vi "Read productId.vi"(8 "error in (no error)":errorcluster, 11 "SCD in":refnum<class "SCD.lvclass">) -> (0 "error out":errorcluster, 2 "productId":i32, 3 "SCD out":refnum<class "SCD.lvclass">)   [LabVIEW 2023, in "SCD.lvclass"]
uses:
  SCD.lvclass
  GenericDevice/GenericDevice.lvclass
panel:
  # "Connector Pane"
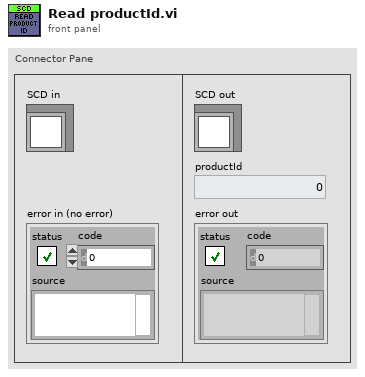
[diagram p1: front panel]
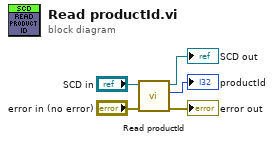
[diagram p0: block diagram]
diagram:
  n1 = call-parent "Read productId.vi"("error in (no error)"="error in (no error)", "GenericDevice in"="SCD in") -> ("error out"=→"error out":errorcluster, "productId"=→"productId":i32, "GenericDevice out"=→"SCD out":refnum<class "SCD.lvclass">)  [unwired: 7 in]
